vi "GaGe4_ConfigureChannels.vi"(8 "error in (no error)":errorcluster, 10 "Input settings":T1(array[cluster]), 11 "Handle Cluster in":T2) -> (0 "error out":errorcluster)   [LabVIEW 2015]
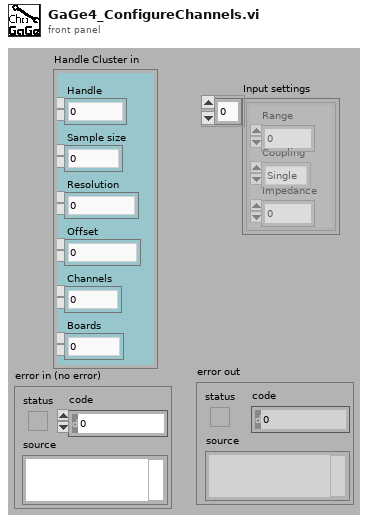
[diagram p1: front panel]
types:
  T1 = cluster{"Range":dbl, "Coupling":enum16{"Single", "Differen"}, "Impedance":dbl}[]
  T2 = cluster{"Handle":u32, "Sample size":u32, "Resolution":i32, "Offset":i32, "Channels":u32, "Boards":u32}
  T3 = cluster{"Coupling":string, bool, "Direct-to-ADC":bool, i32, u32, "DC Offset":i32}
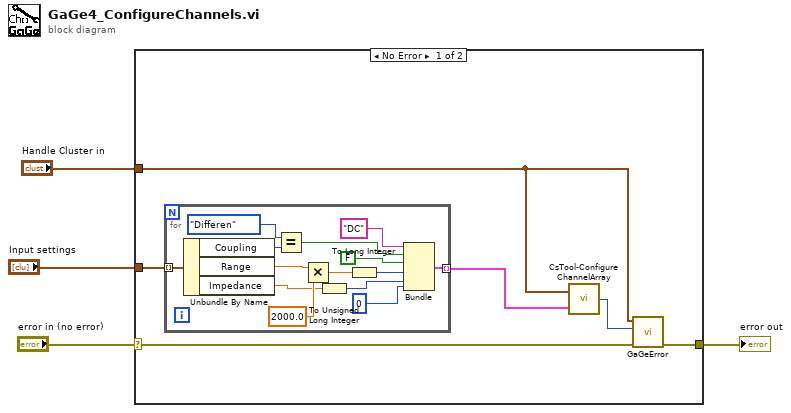
[diagram p0: block diagram]
diagram:
  n1 = case shown="No Error" "error in (no error)" {
    selector: "error in (no error)" -> [w10 w25]
    tunnel: [w9 w25] -> w3
    tunnel: "Handle Cluster in" -> [w8 _]
    tunnel: "Input settings" -> [w6 _]
    frame No Error {
      n2 = for {
        tunnel: w6 -> [w24] mode=indexing
        tunnel: [w15] -> w5 mode=indexing
        n3 = Unbundle By Name(w24) -> ("Coupling"=w18:enum16{"Single", "Differen"}, "Range"=w20:dbl, "Impedance"=w14:dbl)
        n4 = Equal?(x=enum16{"Single", "Differen"}."Differen" ("Coupling"), y=w18) -> (x = y?=w16:bool)
        n5 = Multiply(x=w20, y=2000.0 ("x")) -> (x*y=w23:dbl)
        n6 = To Unsigned Long Integer(number=w14) -> (unsigned 32bit integer=w12:u32)
        n7 = To Long Integer(number=w23) -> (32bit integer=w11:i32)
        n8 = Bundle("Coupling"="DC", w16, "Direct-to-ADC"=FALSE, w11, w12, "DC Offset"=0) -> (w15:T3)  [unwired: 1 out]
      }
      n9 = call "CsTool-ConfigureChannelArray.vi"("Channels"=w5, "Handle Cluster"=w8) -> ("Error Code"=w7:u32)
      n10 = call "GaGeError.vi"("error in (no error)"=w10, "Error Code"=w7, "Handle Cluster"=w8) -> ("error out"=w9:errorcluster)  [unwired: 3 in, 5 out]
    }
    frame Error {
    }
  }
  "error out" <- w3
